vi "Resolve or Create Folder.vi"(8 "Error In":errorcluster, 11 "path (unresolved)":path) -> (0 "Error Out":errorcluster, 3 "path (resolved)":path)   [LabVIEW 2014]
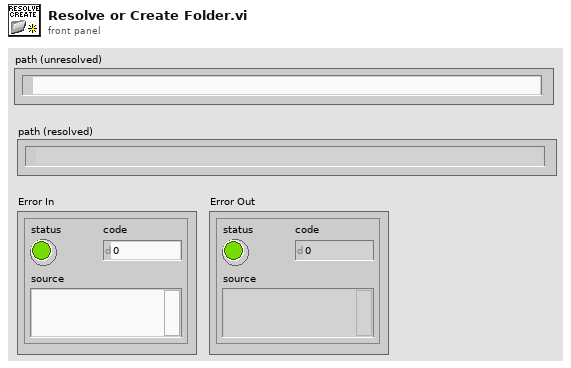
[diagram p1: front panel]
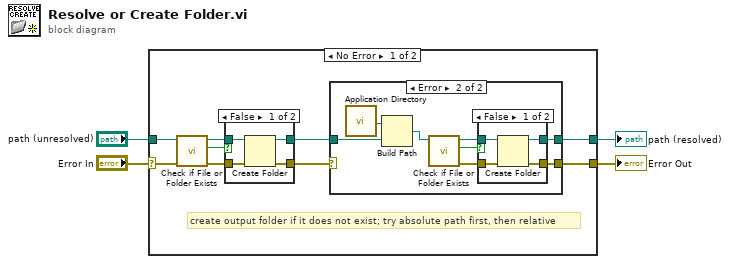
[diagram p0: block diagram]
diagram:
  n1 = case shown="No Error" "Error In" {
    selector: "Error In" -> [w8 w36]
    tunnel: [w5 w37] -> w4
    tunnel: "path (unresolved)" -> [w6 w37]
    tunnel: [w7 w36] -> w1
    frame No Error {
      # "create output folder if it does not exist; try absolute path first, then relative"
      n2 = call <vilib>:"Check if File or Folder Exists.vi"("error in (no error)"=w8, "path"=w6) -> ("error out"=w11:errorcluster, "file or folder exists?"=w12:bool, "dup path"=w13:path)  [unwired: 7 in]
      n3 = case shown="False" w12 {
        tunnel: w11 -> [w33 w34]
        tunnel: w13 -> [w32 w35]
        tunnel: [w31 w35] -> w10
        tunnel: [w30 w34] -> w9
        frame False {
          n4 = Create Folder(path (use dialog)=w32, error in=w33) -> (created path=w31:path, error out=w30:errorcluster)  [unwired: 1 in, 1 out]
        }
        frame True {
        }
      }
      n5 = case shown="Error" w9 {
        selector: w9 -> [w14 _]
        tunnel: [w15 w20] -> w5
        tunnel: w10 -> [w15 w22]
        tunnel: [w14 w19] -> w7
        frame No Error {
        }
        frame Error {
          n6 = call <vilib>:"Application Directory.vi"() -> ("Application Directory"=w23:path)
          n7 = Build Path(base path=w23, name or relative path=w22) -> (appended path=w21:path)
          n8 = call <vilib>:"Check if File or Folder Exists.vi"("path"=w21) -> ("error out"=w17:errorcluster, "file or folder exists?"=w16:bool, "dup path"=w18:path)  [unwired: 8 in]
          n9 = case shown="False" w16 {
            tunnel: w17 -> [w27 w28]
            tunnel: w18 -> [w26 w29]
            tunnel: [w25 w29] -> w20
            tunnel: [w24 w28] -> w19
            frame False {
              n10 = Create Folder(path (use dialog)=w26, error in=w27) -> (created path=w25:path, error out=w24:errorcluster)  [unwired: 1 in, 1 out]
            }
            frame True {
            }
          }
        }
      }
    }
    frame Error {
    }
  }
  "path (resolved)" <- w4
  "Error Out" <- w1
